vi "ABB configure Heat run.vi"() -> ()   [LabVIEW 2017]
uses:
  Temp error msg.ctl
  ABB global.vi
panel:
  in  "Temp error":T1="Error: Temperature measurement "
  in  "x":bool
  in  "Category":T2(ring)
  in  "delete reading":bool
  in  "Add reading":bool
  in  "Temperature Measurement channels":i32(listbox)
  in  "Temperature Readings":i32(listbox)
  in  "Auto Reading":T3={"Thermal Stability (%)"=2.0, "Reading interval (mins)"=2.0}
  in  "Exit":bool
  # "Configure Heat Run"
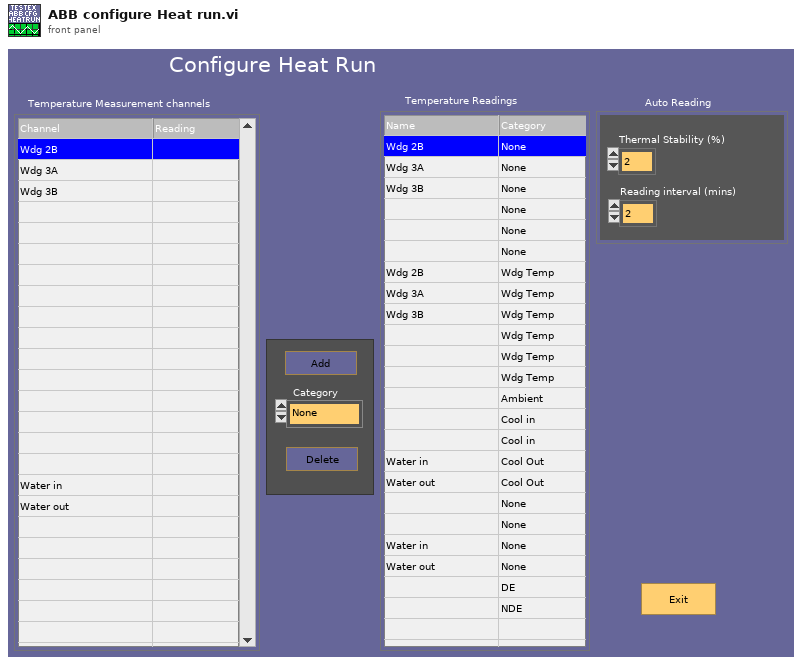
[diagram p1: front panel]
types:
  T1 = typedef "Temp error msg.ctl" = string
  T2 = enum16{"None", "Cool in", "Cool Out", "Wdg Temp", "Ambient", "DE", "NDE", "Aux coolant"}
  T3 = cluster{"Thermal Stability (%)":dbl, "Reading interval (mins)":dbl}
  T4 = cluster{"temp. alloc":i32[], "category":i32[], "Category names":string[], "Category none names":string[]}
  T5 = cluster{"Thermal Stability (deg/hr)":dbl, "Reading interval (mins)":dbl}
  T6 = cluster{"Simulate Norma":bool, "Norma 5000 Address":u8, "WebDaq IP Address":string, "Simulate cDAQ":bool}
  T7 = cluster{"temp. alloc":i32[], "category":i32[], string[], string[]}
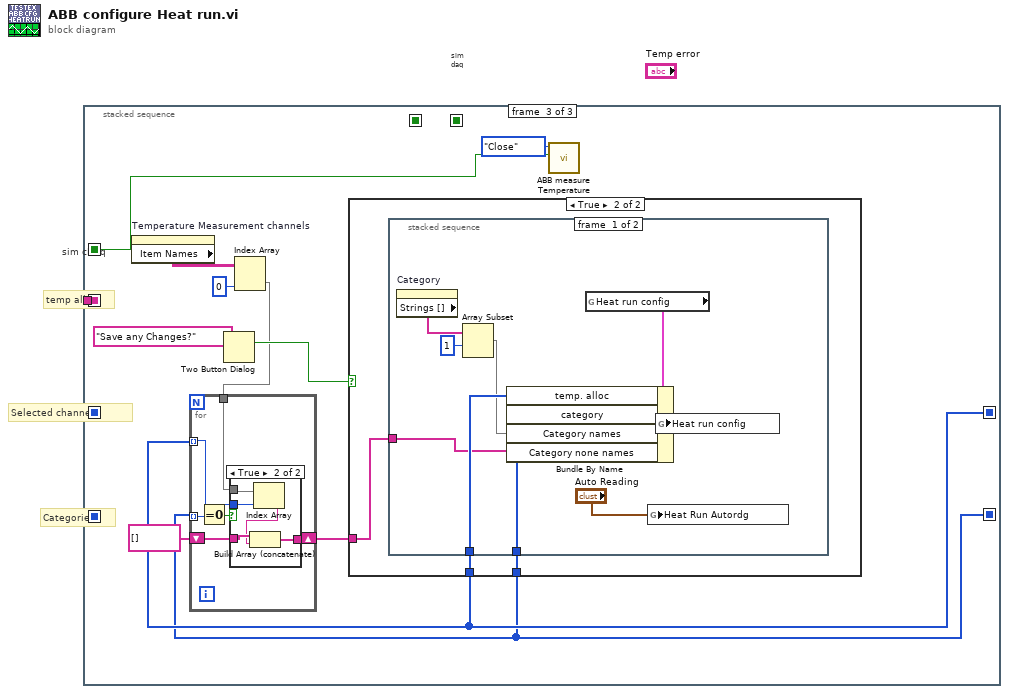
[diagram p0: block diagram]
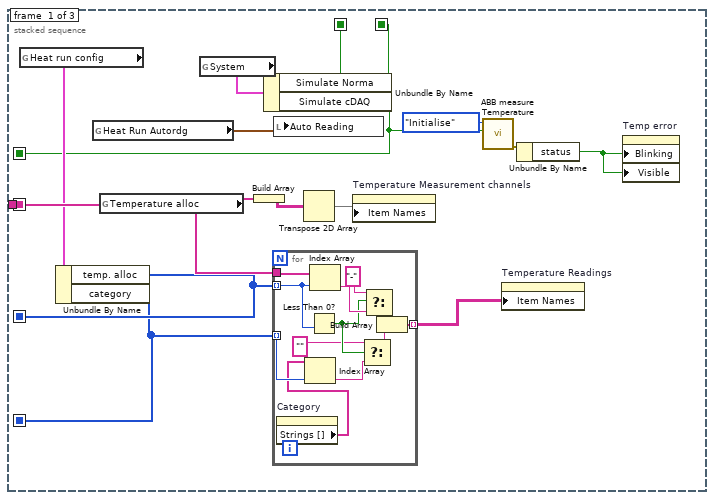
[diagram p2: hidden frame]
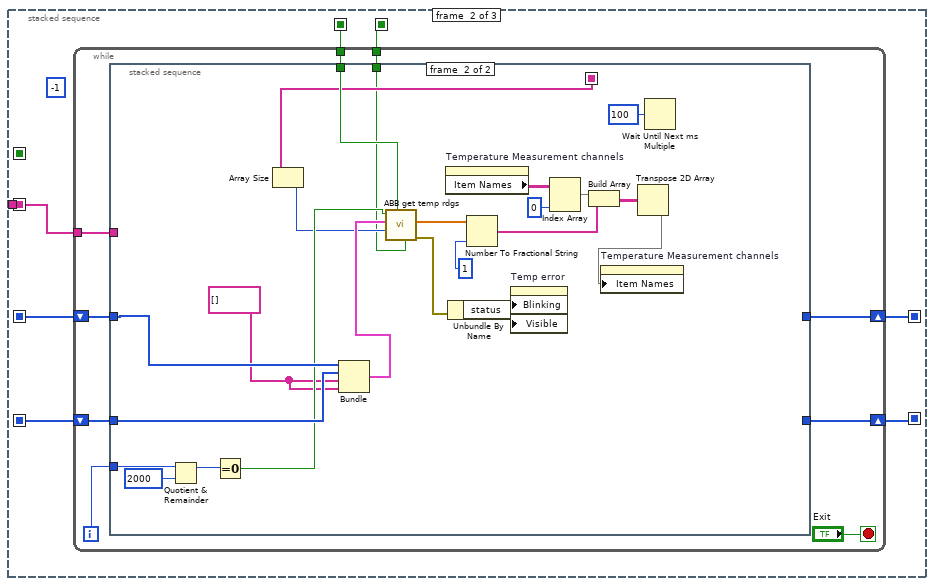
[diagram p3: hidden frame]
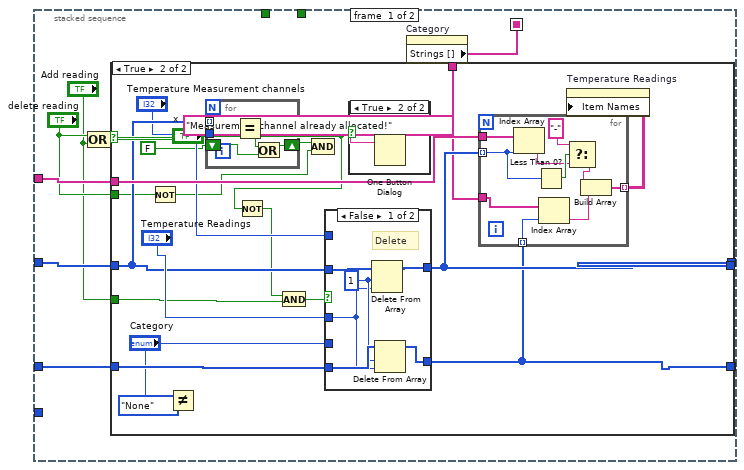
[diagram p4: hidden frame]
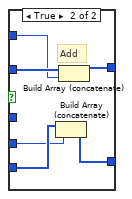
[diagram p7: hidden frame]
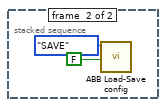
[diagram p10: hidden frame]
diagram:
  # "sim daq"
  # "sim cDaq"
  # "Categories"
  # "Selected channels"
  # "temp alloc"
  n1 = stacked-sequence {
    seq-local: [w8 _ _] -> [_ w33 _]
    seq-local: [_ w32 _] -> [_ _ w127]
    seq-local: [w11 _ _] -> [_ w31 _]
    seq-local: [w7 _ _] -> [_ w30 _]
    seq-local: [_ w29 _] -> [_ _ w126]
    seq-local: [w5 _ _] -> [_ w28 _]
    seq-local: [w3 _ _] -> [_ _ w124]
    seq-local: [w3 _ _] -> [_ w27 _]
    tunnel: [w11 _ _] -> _
    frame #0 {
      n2 = global read "ABB global.vi" "Heat run config"() -> (w10:T4)
      n3 = Unbundle By Name(w10) -> ("temp. alloc"=w8:i32[], "category"=w7:i32[])
      n4 = global read "ABB global.vi" "Heat Run Autordg"() -> (w14:T5)
      n5 = global read "ABB global.vi" "Temperature alloc"() -> (w11:string[])
      n6 = global read "ABB global.vi" "System"() -> (w6:T6)
      n7 = Build Array(w11) -> (w13:string[][])
      n8 = Unbundle By Name(w6) -> ("Simulate Norma"=w5:bool, "Simulate cDAQ"=w3:bool)
      n9 = for {
        tunnel: w11 -> [w26]
        tunnel: w8 -> [w23] mode=indexing
        tunnel: w7 -> [w21] mode=indexing
        tunnel: [w16] -> w9 mode=indexing
        n10 = property on="Category" class="Enum (strict)"() -> ("Strings []"=w20:string[])  [unwired: 2 in, 2 out]
        n11 = Index Array(array=w20, index=w21) -> (element=w19:string)
        n12 = Less Than 0?(x=w23) -> (x < 0?=w22:bool)
        n13 = Index Array(array=w26, index=w23) -> (element=w24:string)
        n14 = Select(t="", s=w22, f=w19) -> (s? t:f=w18:string)
        n15 = Select(t="-", s=w22, f=w24) -> (s? t:f=w17:string)
        n16 = Build Array(w17, w18) -> (w16:string[])
      }
      n17 = local write "Auto Reading"(w14) -> ()
      n18 = Transpose 2D Array(2D array=w13) -> (transposed array=w12:string[][])
      n19 = property on="Temperature Measurement channels" class="MCListbox (strict)"("Item Names"=w12) -> ()  [unwired: 2 in, 2 out]
      n20 = call "ABB measure Temperature.vi"("Simulate"=w3, "Mode"=enum16{"Initialise", "Read", "Close"}."Initialise") -> ("error out"=w2:errorcluster)  [unwired: 7 in, 2 out]
      n21 = property on="Temperature Readings" class="MCListbox (strict)"("Item Names"=w9) -> ()  [unwired: 2 in, 2 out]
      n22 = Unbundle By Name(w2) -> ("status"=w1:bool)
      n23 = property on="Temp error" class="Str (strict)"("Blinking"=w1, "Visible"=w1) -> ()  [unwired: 2 in, 2 out]
    }
    frame #1 {
      (unwired) -1 ("Number Values")
      n24 = while {
        shift-right: [w40] -> w32
        shift-left: w33 -> [w41]
        tunnel: w31 -> [w39]
        shift-right: [w37] -> w29
        shift-left: w30 -> [w38]
        tunnel: w28 -> [w36]
        tunnel: w27 -> [w34]
        i -> [w35]
        stop <- "Exit" stop-if-true
        n25 = stacked-sequence {
          seq-local: [w43 _] -> [_ w105]
          tunnel: w41 -> [w51 w121]
          tunnel: [w50 _] -> w40
          tunnel: w39 -> [w49 _]
          tunnel: w38 -> [w46 w122]
          tunnel: [w45 _] -> w37
          tunnel: w36 -> [_ w123]
          tunnel: w35 -> [_ w110]
          tunnel: w34 -> [_ w103]
          frame #0 {
            n26 = Compound Arithmetic op=OR("delete reading", "Add reading") -> (w48:bool)
            n27 = property on="Category" class="Enum (strict)"() -> ("Strings []"=w43:string[])  [unwired: 2 in, 2 out]
            n28 = case shown="True" w48 {
              tunnel: w51 -> [w53 w66]
              tunnel: [w53 w70] -> w50
              tunnel: w49 -> [_ w72]
              tunnel: "delete reading" -> [_ w60]
              tunnel: w46 -> [w52 w69]
              tunnel: [w52 w68] -> w45
              tunnel: "Add reading" -> [_ w57]
              tunnel: w43 -> [_ w58]
              frame False {
              }
              frame True {
                n29 = Not(x=w60) -> (.not. x?=w59:bool)
                n30 = Not Equal?(x="Category", y=T2."None") -> ()  [unwired: 1 out]
                n31 = for {
                  tunnel: w66 -> [w78] mode=indexing
                  tunnel: "Temperature Measurement channels" -> [w77]
                  shift-right: [w74] -> w62
                  shift-left: FALSE -> [w75]
                  n32 = Equal?(x=w78, y=w77) -> (x = y?=w76:bool)
                  n33 = Or(x=w76, y=w75) -> (x .or. y?=w74:bool)
                }
                n34 = Not(x="x") -> (.not. x?=w61:bool)
                n35 = And(x=w61, y=w57) -> (x .and. y?=w63:bool)
                n36 = Compound Arithmetic op=AND(w62, w59) -> ()  [unwired: 1 out]
                n37 = case shown="False" w63 {
                  tunnel: "Category" -> [_ w86]
                  tunnel: "Temperature Measurement channels" -> [_ w88]
                  tunnel: w66 -> [w84 w90]
                  tunnel: [w83 w89] -> w70
                  tunnel: w69 -> [w82 w87]
                  tunnel: [w81 w85] -> w68
                  tunnel: "Temperature Readings" -> [w79 _]
                  frame False {
                    w80 = 1 ("length")
                    # "Delete"
                    n38 = Delete From Array(array=w84, length=w80, index=w79) -> (array with subset deleted=w83:i32[])  [unwired: 1 out]
                    n39 = Delete From Array(array=w82, length=w80, index=w79) -> (array with subset deleted=w81:i32[])  [unwired: 1 out]
                  }
                  frame True {
                    # "Add"
                    n40 = Build Array (concatenate)(w87, w86) -> (w85:i32[])
                    n41 = Build Array (concatenate)(w90, w88) -> (w89:i32[])
                  }
                }
                n42 = case shown="True" "x" {
                  frame False {
                  }
                  frame True {
                    n43 = One Button Dialog(message="Measurement channel already allocated!") -> ()  [unwired: 1 in, 1 out]
                  }
                }
                n44 = for {
                  tunnel: w70 -> [w99] mode=indexing
                  tunnel: w72 -> [w100]
                  tunnel: w58 -> [w94]
                  tunnel: w68 -> [w95] mode=indexing
                  tunnel: [w91] -> w71 mode=indexing
                  n45 = Index Array(array=w100, index=w99) -> (element=w97:string)
                  n46 = Less Than 0?(x=w99) -> (x < 0?=w98:bool)
                  n47 = Index Array(array=w94, index=w95) -> (element=w92:string)
                  n48 = Select(t="-", s=w98, f=w97) -> (s? t:f=w93:string)
                  n49 = Build Array(w93, w92) -> (w91:string[])
                }
                n50 = property on="Temperature Readings" class="MCListbox (strict)"("Item Names"=w71) -> ()  [unwired: 2 in, 2 out]
              }
            }
          }
          frame #1 {
            w106 = string[] []
            n51 = Quotient & Remainder(x=w110, y=2000) -> (x-y*floor(x/y)=w108:i32)  [unwired: 1 out]
            n52 = Equal To 0?(x=w108) -> (x = 0?=w107:bool)
            n53 = Array Size(array=w105) -> (size(s)=w104:i32)
            n54 = Bundle("temp. alloc"=w121, "category"=w122, w106, w106) -> (w120:T7)  [unwired: 1 in]
            n55 = call "ABB get temp rdgs.vi"("Sim daq"=w103, "Simulate norma"=w123, "# categories"=w104, "run config"=w120, "start"=w107) -> ("error out"=w102:errorcluster, "Measured temps"=w119:dbl[])  [unwired: 3 in, 2 out]
            n56 = property on="Temperature Measurement channels" class="MCListbox (strict)"() -> ("Item Names"=w117:string[][])  [unwired: 2 in, 2 out]
            n57 = Unbundle By Name(w102) -> ("status"=w101:bool)
            n58 = Number To Fractional String(number=w119, precision (6)=i16 1) -> (F-format string=w114:string[])  [unwired: 2 in]
            n59 = property on="Temp error" class="Str (strict)"("Blinking"=w101, "Visible"=w101) -> ()  [unwired: 2 in, 2 out]
            n60 = Index Array(array=w117, index (col)=0 ("disabled index (col)")) -> (element=w115:string[])  [unwired: 1 in]
            n61 = Build Array(w115, w114) -> (w113:string[][])
            n62 = Transpose 2D Array(2D array=w113) -> (transposed array=w112:string[][])
            n63 = property on="Temperature Measurement channels" class="MCListbox (strict)"("Item Names"=w112) -> ()  [unwired: 2 in, 2 out]
            n64 = Wait Until Next ms Multiple(millisecond multiple=u32 100) -> ()  [unwired: 1 out]
          }
        }
      }
    }
    frame #2 {
      n65 = property on="Temperature Measurement channels" class="MCListbox (strict)"() -> ("Item Names"=w132:string[][])  [unwired: 2 in, 2 out]
      n66 = Two Button Dialog(message="Save any Changes?") -> (T button?=w134:bool)  [unwired: 2 in]
      n67 = Index Array(array=w132, index (col)=0 ("disabled index (col)")) -> (element=w130:string[])  [unwired: 1 in]
      n68 = for {
        tunnel: w127 -> [w137] mode=indexing
        tunnel: w126 -> [w139] mode=indexing
        tunnel: w130 -> [w138]
        shift-right: [w135] -> w128
        shift-left: string[] [] -> [w136]
        n69 = Equal To 0?(x=w139) -> (x = 0?=w140:bool)
        n70 = case shown="True" w140 {
          tunnel: w138 -> [_ w146]
          tunnel: w137 -> [_ w145]
          tunnel: [w141 w144] -> w135
          tunnel: w136 -> [w141 w143]
          frame False {
          }
          frame True {
            n71 = Index Array(array=w146, index=w145) -> (element=w142:string)
            n72 = Build Array (concatenate)(w143, w142) -> (w144:string[])
          }
        }
      }
      n73 = case shown="True" w134 {
        tunnel: w127 -> [_ w149]
        tunnel: w126 -> [_ w148]
        tunnel: w128 -> [_ w147]
        frame False {
        }
        frame True {
          n74 = stacked-sequence {
            tunnel: w149 -> [w157 _]
            tunnel: w148 -> [w155 _]
            tunnel: w147 -> [w153 _]
            frame #0 {
              n75 = property on="Category" class="Enum (strict)"() -> ("Strings []"=w151:string[])  [unwired: 2 in, 2 out]
              n76 = Array Subset(array=w151, index=1) -> (w152:string[])  [unwired: 1 in]
              n77 = global read "ABB global.vi" "Heat run config"() -> (w158:T4)
              n78 = Bundle By Name(cluster=w158, "temp. alloc"=w157, "category"=w155, "Category names"=w152, "Category none names"=w153) -> (w156:T4)
              n79 = global write "ABB global.vi" "Heat Run Autordg"("Auto Reading") -> ()
              n80 = global write "ABB global.vi" "Heat run config"(w156) -> ()
            }
            frame #1 {
              n81 = call "ABB Load-Save config.vi"("confirm save"=FALSE, "Mode"=enum16{"LOAD", "SAVE"}."SAVE") -> ()  [unwired: 10 in]
            }
          }
        }
      }
      n82 = call "ABB measure Temperature.vi"("Simulate"=w124, "Mode"=enum16{"Initialise", "Read", "Close"}."Close") -> ()  [unwired: 7 in, 3 out]
    }
  }
